vi "Get VS Direction.vi"(8 "error in (no error)":errorcluster, 10 "Modbus Type":T2, 11 "Item Ref in":T1 format="%.0x") -> (0 "error out":errorcluster, 2 "Veristand Type":T3, 3 "Item Ref out":T1 format="%.0x")   [LabVIEW 2015, in "Modbus Master System Explorer.lvlib"]
uses:
  Modbus Master System Explorer.lvlib
  <vilib>/NI Veristand/Custom Device API/Custom Device Channel Type.ctl
  Modbus Type.ctl
  <vilib>/NI Veristand/Custom Device API/Custom Device Item Ref.ctl
  <vilib>/NI VeriStand/Custom Device API/Custom Device API.lvlib
  Shared/Modbus Master Shared.lvlib
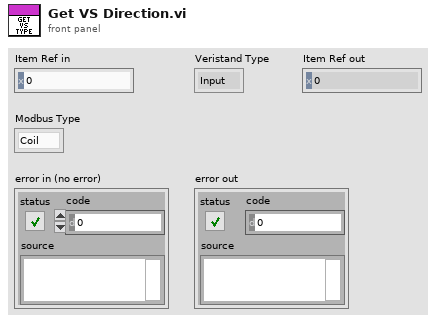
[diagram p1: front panel]
types:
  T1 = typedef "Custom Device API.lvlib/Custom Device Item Ref.ctl" = u64
  T2 = typedef "Modbus Master Shared.lvlib/Modbus Type.ctl" = enum16{"Coil", "Discrete Input", "Holding Register", "Input Register"}
  T3 = typedef "Custom Device API.lvlib/Custom Device Channel Type.ctl" = enum16{"Input", "Output"}
  T4 = typedef "Modbus Master Shared.lvlib/Interface Type.ctl" = enum16{"TCP Master", "Serial Master"}
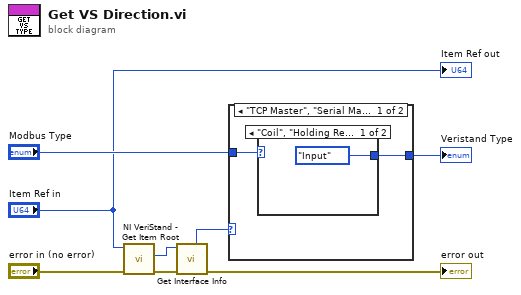
[diagram p0: block diagram]
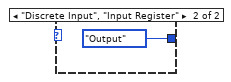
[diagram p2: hidden frame]
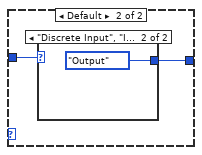
[diagram p3: hidden frame]
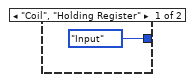
[diagram p4: hidden frame]
diagram:
  n1 = call <vilib>:"NI VeriStand - Get Item Root.vi"("error in (no error)"="error in (no error)", "Item Ref in"="Item Ref in") -> ("error out"=w4:errorcluster, "Root Ref out"=w5:T1)  [unwired: 6 in, 2 out]
  n2 = call "Get Interface Info.vi"("error in (no error)"=w4, "Device Item Ref in"=w5) -> ("error out"=→"error out":errorcluster, "Interface Type"=w6:T4)  [unwired: 4 in, 4 out]
  n3 = case shown="\"TCP Master\", \"Serial Master\"" w6 {
    tunnel: "Modbus Type" -> [w10 w13]
    tunnel: [w9 w14] -> w8
    frame "TCP Master", "Serial Master" {
      n4 = case shown="\"Coil\", \"Holding Register\"" w10 {
        tunnel: [Custom_Device_Channel_Type."Input" ("Veristand Type") Custom_Device_Channel_Type."Output" ("Veristand Type")] -> w9
        frame "Coil", "Holding Register" {
        }
        frame "Discrete Input", "Input Register" {
        }
      }
    }
    frame Default {
      n5 = case shown="\"Discrete Input\", \"Input Register\"" w13 {
        tunnel: [Custom_Device_Channel_Type."Input" ("Veristand Type") Custom_Device_Channel_Type."Output" ("Veristand Type")] -> w14
        frame "Coil", "Holding Register" {
        }
        frame "Discrete Input", "Input Register" {
        }
      }
    }
  }
  "Veristand Type" <- w8
  "Item Ref out" <- "Item Ref in"
